vi "Write KickY.vi"(8 "error in (no error)":errorcluster, 10 "KickY":dbl, 11 "KickToSkill in":refnum<class "KickToSkill.lvclass">) -> (0 "error out":errorcluster, 3 "KickToSkill out":refnum<class "KickToSkill.lvclass">)   [LabVIEW 2023]
uses:
  KickToSkill.lvclass
  C:/Users/ebert/Desktop/roboime/SSL_AI/Skill_class/Skill.lvclass
  C:/Users/ebert/Desktop/roboime/SSL_AI/KickToSkill_class/KickToSkill.lvclass
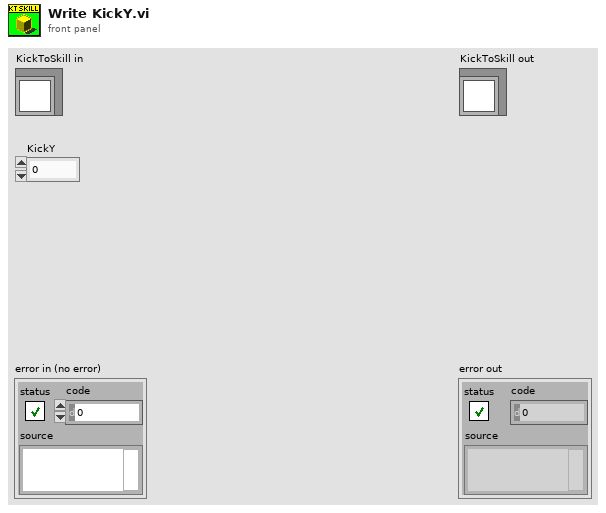
[diagram p1: front panel]
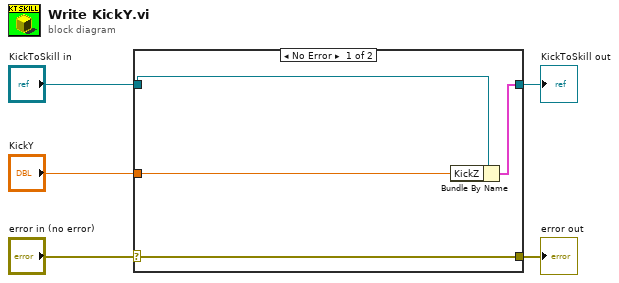
[diagram p0: block diagram]
diagram:
  n1 = case shown="No Error" "error in (no error)" {
    selector: "error in (no error)" -> [w9 w10]
    tunnel: [w9 w10] -> w4
    tunnel: [w7 w11] -> w2
    tunnel: "KickToSkill in" -> [w8 w11]
    tunnel: "KickY" -> [w6 _]
    frame No Error {
      n2 = Bundle By Name(cluster=w8, "KickZ"=w6) -> (w7:cluster{})
    }
    frame Error {
    }
  }
  "error out" <- w4
  "KickToSkill out" <- w2
